vi "xps_generate_dither_pvt_trajectory.vi"(7 "Dither Cycles":u32=3, 8 "error in (no error)":errorcluster, 9 "custom?":bool=TRUE, 10 "Custom Dither Trajectory":T1 {"Dither Period (s)" min=0.0; "PVT Ampl (nm)" min=0.0}, 11 "newport_xps in":refnum<class "newport_xps.lvclass">) -> (0 "error out":errorcluster, 3 "newport_xps out":refnum<class "newport_xps.lvclass">)   [LabVIEW 2015, in "newport_xps.lvclass"]
uses:
  newport_xps.lvclass
  dither_trajectory_settings.ctl
  dither_trajectory_types.ctl
  newport_xps.lvclass/newport_xps.ctl
  <vilib>/Utility/file.llb/Write Delimited Spreadsheet (DBL).vi
  <vilib>/FTP/NI_FTP.lvlib
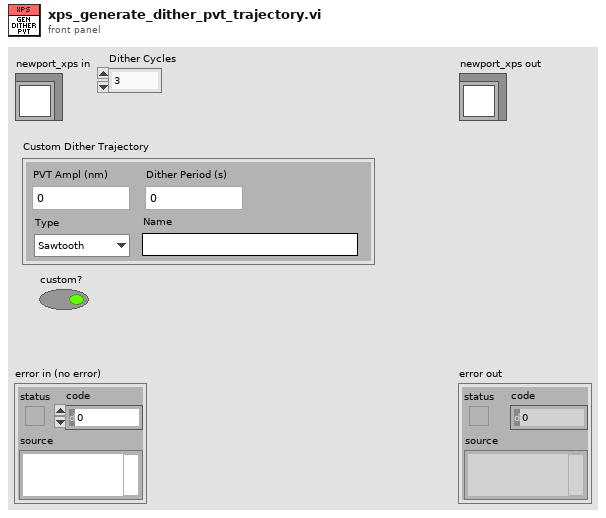
[diagram p1: front panel]
types:
  T1 = typedef "dither_trajectory_settings.ctl" = cluster{"PVT Ampl (nm)":dbl, "Dither Period (s)":dbl, "Type":T2, "Name":string}
  T2 = typedef "dither_trajectory_types.ctl" = enum16{"Sawtooth"}
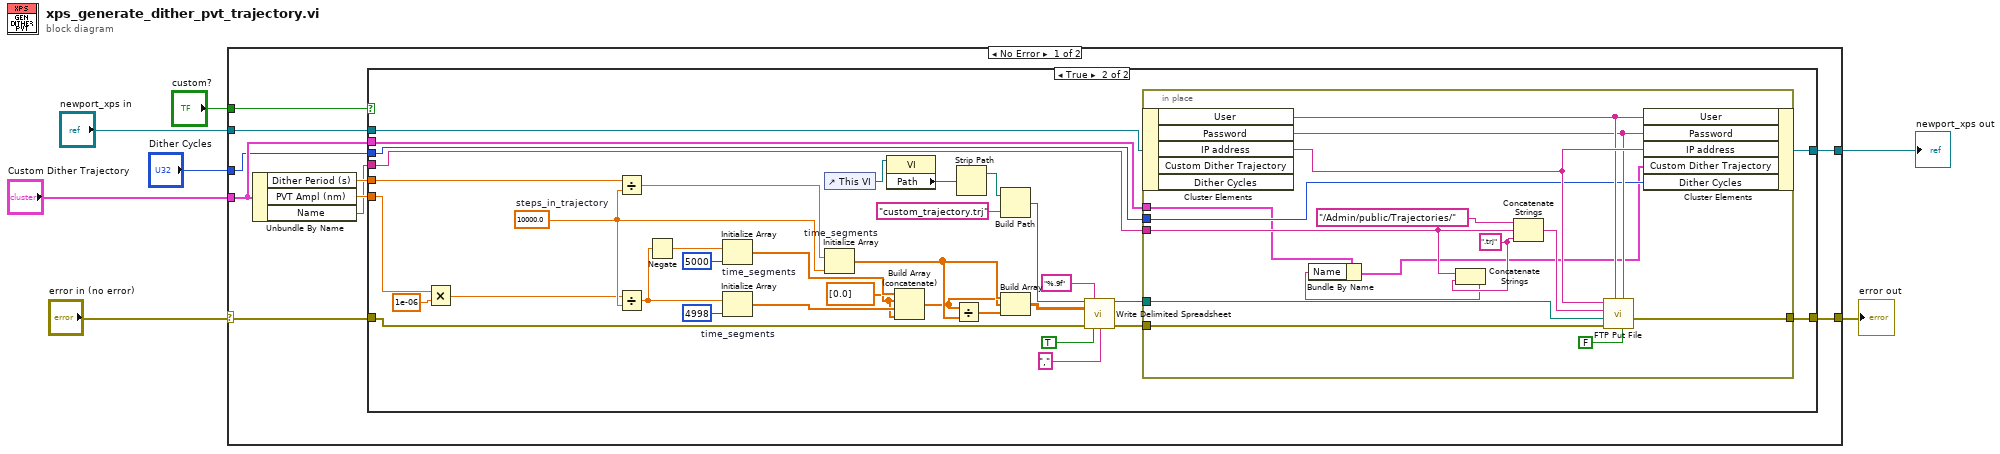
[diagram p0: block diagram]
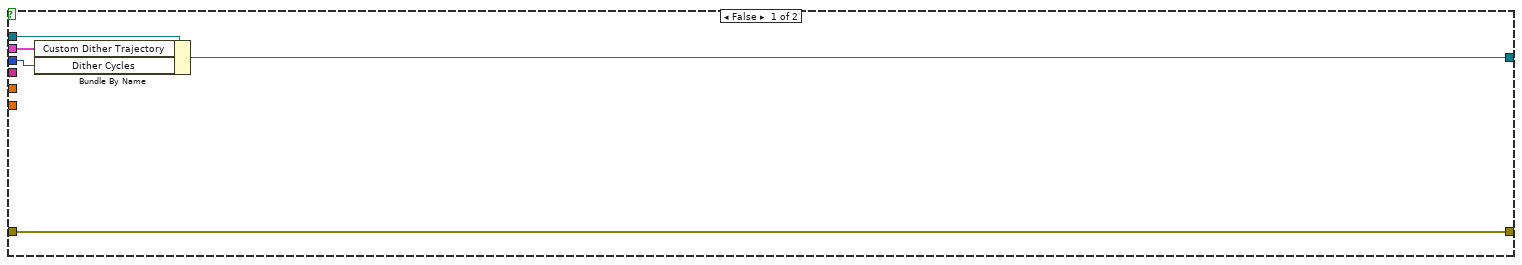
[diagram p2: hidden frame]
diagram:
  n1 = case shown="No Error" "error in (no error)" {
    selector: "error in (no error)" -> [w13 w73]
    tunnel: [w12 w73] -> w6
    tunnel: "newport_xps in" -> [w15 w72]
    tunnel: "Custom Dither Trajectory" -> [w10 _]
    tunnel: [w14 w72] -> w3
    tunnel: "custom?" -> [w9 _]
    tunnel: "Dither Cycles" -> [w8 _]
    frame No Error {
      n2 = Unbundle By Name(w10) -> ("Dither Period (s)"=w17:dbl, "PVT Ampl (nm)"=w16:dbl, "Name"=w11:string)
      n3 = case shown="True" w9 {
        tunnel: w17 -> [_ w56]
        tunnel: w16 -> [_ w45]
        tunnel: w15 -> [w22 w37]
        tunnel: [w20 w35] -> w14
        tunnel: w13 -> [w19 w34]
        tunnel: [w19 w29] -> w12
        tunnel: w11 -> [_ w28]
        tunnel: w10 -> [w21 w27]
        tunnel: w8 -> [w18 w26]
        frame False {
          n4 = Bundle By Name(cluster=w22, "Custom Dither Trajectory"=w21, "Dither Cycles"=w18) -> (w20:refnum<class "newport_xps.lvclass">)
        }
        frame True {
          w23 = dbl[] [0.0] ("element")
          w54 = 10000.0  # steps_in_trajectory
          n5 = Multiply(x=w45, y=1e-06) -> (x*y=w44:dbl)
          n6 = Divide(x=w56, y=w54) -> (x/y=w55:dbl)
          n7 = Divide(x=w44, y=w54) -> (x/y=w51:dbl)
          n8 = Negate(x=w51) -> (-x=w50:dbl)
          n9 = Initialize Array "time_segments"(w50, 5000 ("dimension size")) -> (w49:dbl[])
          n10 = Initialize Array "time_segments"(w51, 4998 ("dimension size")) -> (w48:dbl[])
          n11 = control-ref of="This VI"() -> (w43:refnum<vi>)
          n12 = Initialize Array "time_segments"(w55, w54) -> (w47:dbl[])
          n13 = property class="VI"(reference=w43) -> ("Path"=w32:path)  [unwired: 1 in, 2 out]
          n14 = Build Array (concatenate)(w49, w23, w48, w23) -> (w25:dbl[])
          n15 = Divide(x=w25, y=w47) -> (x/y=w24:dbl[])
          n16 = Strip Path(path=w32) -> (stripped path=w31:path)  [unwired: 1 out]
          n17 = Build Path(base path=w31, name or relative path="custom_trajectory.trj") -> (appended path=w41:path)
          n18 = Build Array(w47, w25, w24) -> (w40:dbl[][])
          n19 = call-poly <vilib>:"Write Delimited Spreadsheet.vi"("file path (dialog if empty)"=w41, "format (%.3f)"="%.9f", "2D data"=w40, "error in (no error)"=w34, "transpose? (F)"=TRUE, "delimiter (\\t)"="," ("delimiter (\\t)")) -> ("new file path (Not A Path if cancelled)"=w36:path, "error out"=w33:errorcluster)  [unwired: 8 in]
          n20 = in-place {
            in-place-border: w33 -> [w71]
            in-place-border: w36 -> [w66]
            in-place-border: [w70] -> w29
            in-place-border: w28 -> [w61]
            in-place-border: w27 -> [w59]
            in-place-border: w26 -> [w62]
            w60 = ".trj" ("string")
            n21 = in-place-cluster #1(w37) -> ("User"=w68:string, "Password"=w67:string, "IP address"=w69:string)  [unwired: 2 out]
            n22 = Concatenate Strings(w61, w60) -> (w58:string)
            n23 = Bundle By Name(cluster=w59, "Name"=w58) -> (w57:T1)
            n24 = Concatenate Strings("/Admin/public/Trajectories/" ("string"), w61, w60) -> (w63:string)
            n25 = call <vilib>:"FTP Put File.vi"("active (T)"=FALSE, "password"=w67, "user"=w68, "error in (no error)"=w71, "local path"=w66, "remote path"=w63, "host"=w69) -> ("file error"=w70:errorcluster)  [unwired: 3 in, 1 out]
            n26 = in-place-cluster #1("User"=w68, "Password"=w67, "IP address"=w69, "Custom Dither Trajectory"=w57, "Dither Cycles"=w62) -> (w35:refnum<class "newport_xps.lvclass">)
          }
        }
      }
    }
    frame Error {
    }
  }
  "error out" <- w6
  "newport_xps out" <- w3
